vi "Write REM IO VARs.vi"(7 "R/W Case":T7, 8 "error in (no error)":errorcluster, 9 "Input FIFO buffer in":dbl[](array[numeric]), 10 "I/O Input Data In":T1 {"BD Refs"."Data Reference" format="%.0x"}, 11 "I/O Imput Vars in":T4[](array[typedef]) {"VS ref" format="%.0x"}) -> (0 "error out":errorcluster, 1 "Input FIFO buffer out":dbl[](array[numeric]), 2 "I/O Input Data Out":T1 {"BD Refs"."Data Reference" format="%.0x"}, 3 "I/O Imput Vars out":T4[](array[typedef]) {"VS ref" format="%.0x"})   [LabVIEW 2019, in "SEECD Engine.lvlib"]
uses:
  SEECD Engine.lvlib
  Type Defs/RW Case.ctl
  Type Defs/REM IO ECAT Slave IOV Cluster.ctl
  <vilib>/NI VeriStand/Custom Device API/Custom Device Item Ref.ctl
  Type Defs/UDV Data Type.ctl
  Type Defs/Input Data.ctl
  <vilib>/NI VeriStand/Custom Device API/Block Data Reference.ctl
  <vilib>/NI VeriStand/Custom Device API/Data Reference.ctl
  <vilib>/NI VeriStand/Custom Device API/Global Data Refs.vi
  <vilib>/NI VeriStand/Custom Device API/Custom Device API.lvlib
  <vilib>/NI VeriStand/Custom Device Tools/Custom Device Utility Library/Custom Device Utility Library.lvlib
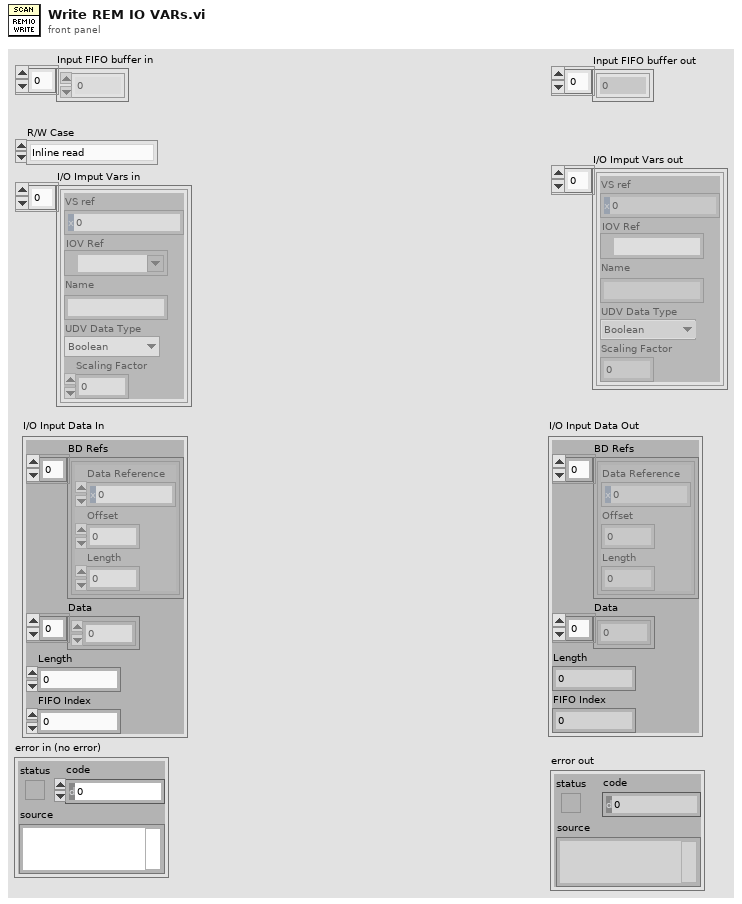
[diagram p1: front panel]
types:
  T1 = typedef "SEECD Engine.lvlib/Input Data.ctl" = cluster{"BD Refs":T2[], "Data":dbl[], "Length":i32, "FIFO Index":i32}
  T2 = typedef "Custom Device API.lvlib/Block Data Reference.ctl" = cluster{"Data Reference":T3, "Offset":u64, "Length":u64}
  T3 = typedef "Custom Device API.lvlib/Data Reference.ctl" = i32
  T4 = typedef "SEECD Engine.lvlib/REM IO ECAT Slave IOV Cluster.ctl" = cluster{"VS ref":T5, "IOV Ref":refnum<k21>, "Name":string, "UDV Data Type":T6, "Scaling Factor":dbl}
  T5 = typedef "Custom Device API.lvlib/Custom Device Item Ref.ctl" = u64
  T6 = typedef "SEECD Engine.lvlib/UDV Data Type.ctl" = enum16{"Boolean", "Fixed Point", "Int8", "Int16", "Int32", "Int64", "U32 Bit Field", "UInt8", "UInt16", "UInt32", "UInt64", "Other", "DBL", "SGL"}
  T7 = typedef "SEECD Engine.lvlib/RW Case.ctl" = enum16{"Inline read", "Inline write", "Async - Inline loop read", "Async - Inline loop write", "Async loop (read/write)"}
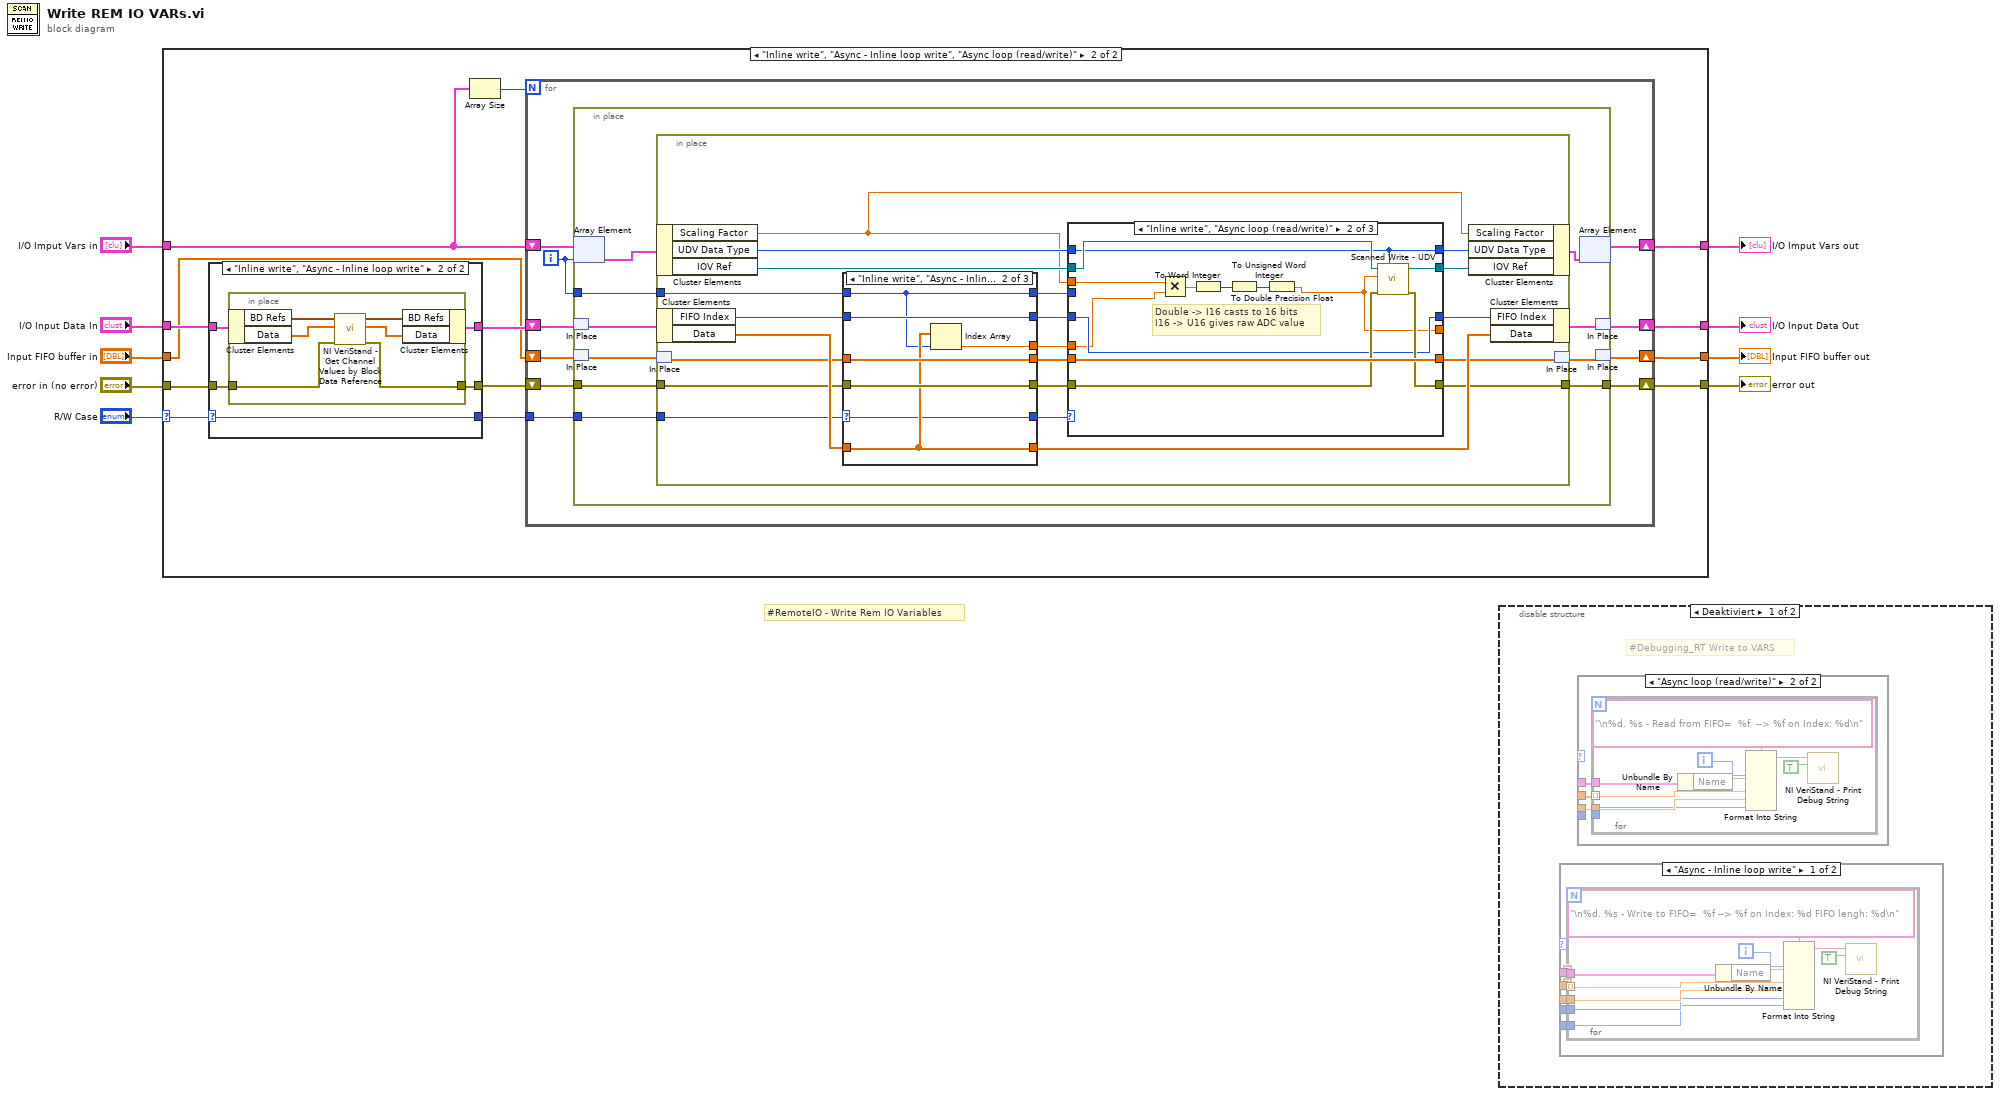
[diagram p0: block diagram]
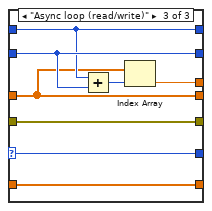
[diagram p4: hidden frame]
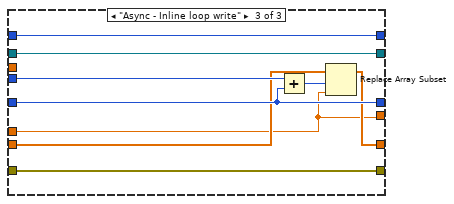
[diagram p6: hidden frame]
diagram:
  # "#RemoteIO - Write Rem IO Variables"
  n1 = case shown="\"Inline write\", \"Async - Inline loop write\", \"Async loop (read/write)\"" "R/W Case" {
    selector: "R/W Case" -> [_ w22]
    tunnel: [w11 w26] -> w5
    tunnel: "Input FIFO buffer in" -> [w11 w14]
    tunnel: [w12 w16] -> w2
    tunnel: [w13 w25] -> w6
    tunnel: "I/O Input Data In" -> [w12 w20]
    tunnel: "I/O Imput Vars in" -> [w13 w24]
    tunnel: [w10 w15] -> w4
    tunnel: "error in (no error)" -> [w10 w21]
    frame Default {
    }
    frame "Inline write", "Async - Inline loop write", "Async loop (read/write)" {
      n2 = case shown="\"Inline write\", \"Async - Inline loop write\"" w22 {
        selector: w22 -> [w117 w120]
        tunnel: w20 -> [w118 w124]
        tunnel: w21 -> [w119 w123]
        tunnel: [w119 w122] -> w18
        tunnel: [w118 w121] -> w19
        tunnel: [w117 w120] -> w17
        frame Default {
        }
        frame "Inline write", "Async - Inline loop write" {
          n3 = in-place {
            in-place-border: w123 -> [w126]
            in-place-border: [w125] -> w122
            n4 = in-place-cluster #1(w124) -> ("BD Refs"=w130:T2[], "Data"=w128:dbl[])
            n5 = call <vilib>:"NI VeriStand - Get Channel Values by Block Data Reference.vi"("error in (no error)"=w126, "Values Array in"=w128, "Block Data Ref"=w130) -> ("error out"=w125:errorcluster, "Values Array out"=w127:dbl[], "Block Data Ref dup"=w129:T2[])  [unwired: 6 in]
            n6 = in-place-cluster #1("BD Refs"=w129, "Data"=w127) -> (w121:T1)
          }
        }
      }
      n7 = Array Size(array=w24) -> (size(s)=w23:i32)
      n8 = for {
        N: w23 -> [_]
        shift-right: [w35] -> w25
        shift-left: w24 -> [w36]
        shift-right: [w27] -> w16
        shift-left: w19 -> [w30]
        shift-right: [w33] -> w26
        shift-left: w14 -> [w34]
        shift-right: [w31] -> w15
        shift-left: w18 -> [w32]
        tunnel: w17 -> [w29]
        i -> [w28]
        n9 = in-place {
          in-place-border: w32 -> [w44]
          in-place-border: [w38] -> w31
          in-place-border: w29 -> [w43]
          in-place-border: w28 -> [w42]
          n10 = in-place-array #2(w36, w28) -> (w37:T4)
          n11 = in-place-match #3(w30) -> (w46:T1)
          n12 = in-place-match #4(w34) -> (w45:dbl[])
          n13 = in-place {
            in-place-border: w44 -> [w51]
            in-place-border: w43 -> [w55]
            in-place-border: w42 -> [w66]
            in-place-border: [w49] -> w38
            n14 = in-place-cluster #5(w37) -> ("Scaling Factor"=w48:dbl, "UDV Data Type"=w53:T6, "IOV Ref"=w61:refnum<k21>)
            n15 = in-place-cluster #6(w46) -> ("FIFO Index"=w52:i32, "Data"=w67:dbl[])
            n16 = in-place-match #7(w45) -> (w57:dbl[])
            n17 = case shown="\"Inline write\", \"Async - Inline loop write\"" w55 {
              selector: w55 -> [w70 w75 w84]
              tunnel: w66 -> [w68 w76 w85]
              tunnel: w52 -> [w73 w78 w86]
              tunnel: w57 -> [w71 w79 w83]
              tunnel: w51 -> [w69 w80 w88]
              tunnel: w67 -> [w72 w77 w87]
              tunnel: [w73 w78 w86] -> w62
              tunnel: [w72 w77 w87] -> w58
              tunnel: [w69 w80 w88] -> w50
              tunnel: [w71 w79 w83] -> w54
              tunnel: [w70 w75 w84] -> w60
              tunnel: [_ w74 w82] -> w47
              tunnel: [w68 w76 w85] -> w59
              frame Default {
              }
              frame "Inline write", "Async - Inline loop write" {
                n18 = Index Array(array=w77, index=w76) -> (element=w74:dbl)
              }
              frame "Async loop (read/write)" {
                n19 = Add(x=w85, y=w86) -> (x+y=w81:i32)
                n20 = Index Array(array=w83, index=w81) -> (element=w82:dbl)
              }
            }
            n21 = case shown="\"Inline write\", \"Async loop (read/write)\"" w60 {
              tunnel: w53 -> [w90 w98 w116]
              tunnel: w61 -> [w91 w100 w111]
              tunnel: w62 -> [w92 w103 w113]
              tunnel: w54 -> [w93 w107 w112]
              tunnel: [w93 w107 w110] -> w56
              tunnel: w59 -> [_ _ w114]
              tunnel: [w92 w103 w113] -> w63
              tunnel: [w91 w106 w111] -> w64
              tunnel: [w90 w98 w116] -> w65
              tunnel: w50 -> [w94 w105 w115]
              tunnel: [w94 w104 w115] -> w49
              tunnel: w47 -> [w89 w101 w108]
              tunnel: w48 -> [_ w102 _]
              tunnel: [w89 w99 w108] -> _
              frame Default {
              }
              frame "Inline write", "Async loop (read/write)" {
                # "Double -> I16 casts to 16 bits\nI16 -> U16 gives raw ADC value"
                n22 = Multiply(x=w102, y=w101) -> (x*y=w97:dbl)
                n23 = To Word Integer(number=w97) -> (16bit integer=w96:i16)
                n24 = To Unsigned Word Integer(number=w96) -> (unsigned 16bit integer=w95:u16)
                n25 = To Double Precision Float(number=w95) -> (double precision float=w99:dbl)
                n26 = call "Scanned Write - UDV.vi"("UDV Data Type"=w98, "error in (no error)"=w105, "data in"=w99, "IOV ref in"=w100) -> ("error out"=w104:errorcluster, "IOV ref out"=w106:refnum<k21>)  [unwired: 6 in]
              }
              frame "Async - Inline loop write" {
                n27 = Add(x=w114, y=w113) -> (x+y=w109:i32)
                n28 = Replace Array Subset(array=w112, new element=w108, index=w109) -> (w110:dbl[])
              }
            }
            n29 = in-place-cluster #5("Scaling Factor"=w48, "UDV Data Type"=w65, "IOV Ref"=w64) -> (w41:T4)
            n30 = in-place-cluster #6("FIFO Index"=w63, "Data"=w58) -> (w40:T1)
            n31 = in-place-match #7(w56) -> (w39:dbl[])
          }
          n32 = in-place-array #2(w41) -> (w35:T4[])  [unwired: 1 out]
          n33 = in-place-match #3(w40) -> (w27:T1)
          n34 = in-place-match #4(w39) -> (w33:dbl[])
        }
      }
    }
  }
  "Input FIFO buffer out" <- w5
  "error out" <- w4
  "I/O Imput Vars out" <- w6
  "I/O Input Data Out" <- w2
  n35 = disable-structure shown="Deaktiviert" {
    frame Disabled {
      # "#Debugging_RT Write to VARS"
      n36 = case shown="\"Async - Inline loop write\"" {
        selector: _ -> [_ _]
        tunnel: _ -> [w148 _]
        tunnel: _ -> [w147 _]
        tunnel: _ -> [w146 _]
        tunnel: _ -> [w145 _]
        tunnel: _ -> [w144 _]
        frame "Async - Inline loop write" {
          n37 = for {
            tunnel: w148 -> [w154]
            tunnel: w147 -> [w153] mode=indexing
            tunnel: w146 -> [w151]
            tunnel: w145 -> [w150]
            tunnel: w144 -> [w149]
            i -> [w156]
            n38 = Unbundle By Name(w154) -> ("Name"=w155)
            n39 = Format Into String(format string="\n%d. %s - Write to FIFO=  %f --> %f on Index: %d FIFO lengh: %d\n" ("Format-String"), w156, w155, w153, w151, w150, w149) -> (resulting string=w157:string)  [unwired: 2 in, 1 out]
            n40 = call <vilib>:"NI VeriStand - Print Debug String.vi"("Add to log file? (F)"=TRUE, "Message"=w157) -> ()  [unwired: 9 in, 1 out]
          }
        }
        frame Default {
        }
      }
      n41 = case shown="\"Async loop (read/write)\"" {
        selector: _ -> [_ _]
        tunnel: _ -> [_ w134]
        tunnel: _ -> [_ w133]
        tunnel: _ -> [_ w132]
        tunnel: _ -> [_ w131]
        frame "Async - Inline loop write", Default {
        }
        frame "Async loop (read/write)" {
          n42 = for {
            tunnel: w134 -> [w138]
            tunnel: w133 -> [w137] mode=indexing
            tunnel: w132 -> [w136]
            tunnel: w131 -> [w135]
            i -> [w140]
            n43 = Unbundle By Name(w138) -> ("Name"=w139)
            n44 = Format Into String(format string="\n%d. %s - Read from FIFO=  %f  --> %f on Index: %d\n" ("Format-String"), w140, w139, w137, w136, w135) -> (resulting string=w141:string)  [unwired: 2 in, 1 out]
            n45 = call <vilib>:"NI VeriStand - Print Debug String.vi"("Add to log file? (F)"=TRUE, "Message"=w141) -> ()  [unwired: 9 in, 1 out]
          }
        }
      }
    }
    frame Enabled {
    }
  }
